vi "Get Header By Name.vi"(8 "error in (no error)":errorcluster, 10 "Name":string, 11 "REST Client Headers_NET in":refnum<class "REST Client Headers_NET.lvclass">) -> (0 "error out":errorcluster, 1 "Found?":bool, 2 "Value":string, 3 "REST Client Headers_NET out":refnum<class "REST Client Headers_NET.lvclass">)   [LabVIEW 2018, in "REST Client_NET.lvlib" / "REST Client Headers_NET.lvclass"]
doc: "Get a HTTP response header value by name.\n\nThe VI provides the following arguments.\n\n<b>Name</b> specifies the name of the HTTP header to get."
uses:
  REST Client Headers_NET.lvclass
  REST Client Headers_NET.lvclass/REST Client Headers_NET.ctl
  HttpHeaders_content/HttpHeaders_Content.lvclass
  C:/Viviota/Projects/R&D/LabVIEW_HTTP_REST_NET/HTTPHeaders_NET/HttpHeaders_NET.lvclass
  HttpHeaders_response/HttpHeaders_Response.lvclass
  HTTPHeaders_NET/HttpHeaders_NET.lvclass
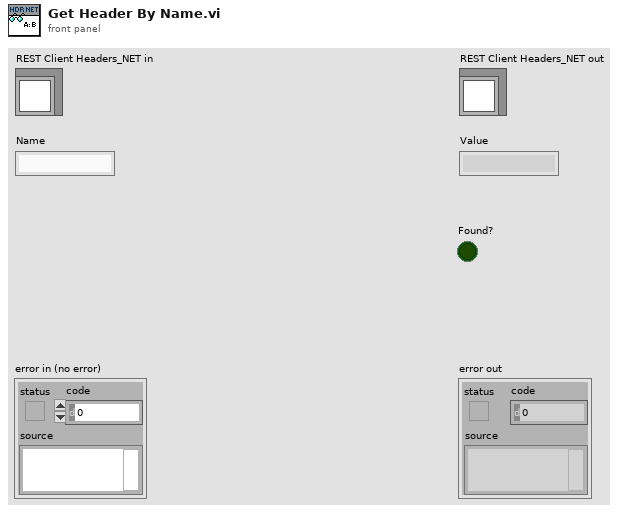
[diagram p1: front panel]
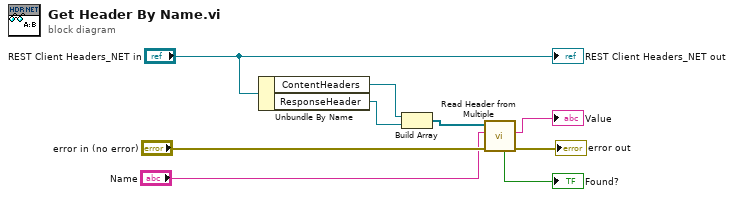
[diagram p0: block diagram]
diagram:
  n1 = Unbundle By Name("REST Client Headers_NET in") -> ("ContentHeaders"=w7:refnum<class "HttpHeaders_Content.lvclass">, "ResponseHeader"=w8:refnum<class "HttpHeaders_Response.lvclass">)
  n2 = Build Array(w7, w8) -> (w3:refnum<class "HttpHeaders_NET.lvclass">[])
  n3 = call "Read Header from Multiple.vi"("error in"="error in (no error)", "Name"="Name", "Headers"=w3) -> ("error out"=→"error out":errorcluster, "Value"=→"Value":string, "Found"=→"Found?":bool)  [unwired: 6 in]
  "REST Client Headers_NET out" <- "REST Client Headers_NET in"
